vi "ScriptsCore.vi"(8 "error in (no error)":errorcluster, 10 "ScriptDatabase":refnum<class "ScriptDatabase.lvclass">, 11 "ScriptsConfiguration":refnum<class "ScriptSetting.lvclass">) -> (0 "error out":errorcluster, 3 "ScriptsConfiguration out":refnum<class "ScriptSetting.lvclass">)   [LabVIEW 2015, in "ScriptSetting.lvclass"]
uses:
  <vilib>/LazyBootMenu/ScriptsConfiguration/ScriptSetting.lvclass
  <vilib>/LazyBootMenu/_Database/Implements/ScriptDatabase.lvclass
  <vilib>/LazyBootMenu/ScriptsConfiguration/Type Definitions/Main Controls and VI Ref in ScriptsConfiguration.ctl
  <vilib>/LazyBootMenu/QDSearchList/QDDialogList.lvclass
  <vilib>/LazyBootMenu/ScriptsConfiguration/ScriptSetting.lvclass/ScriptSetting.ctl
  <vilib>/addons/database/Auxilliary.llb/DB Tools Column Info.ctl
  <vilib>/addons/database/Auxilliary.llb/DB Tools DataTypes.ctl
  <vilib>/LazyBootMenu/_Database/Implements/ScriptDatabase.lvclass/ScriptDatabase.ctl
  <vilib>/Utility/error.llb/Error Cluster From Error Code.vi
  <vilib>/ErrorRing/Error Ring.xnode
  <vilib>/LazyBootMenu/_Database/Ancestor/DatabaseAPI.lvclass
  <vilib>/addons/database/NI_Database_API.lvlib
panel:
  in  "Operation Tab":enum32{"QDFunctions", "Setting", "Options"}(tab)
  in  "Remove Select Shortcut(s)":bool
  in  "Add":bool
  in  "QD Function Full Name":string(combo)
  in  "QDAcroynm":string
  in  "QDFunction Shortcuts":i32[](listbox)
  in  "Import Shortcuts Configuration File":bool
  in  "QDFunction Library Path":path
  in  "Fresh":bool caption="Fresh QD Library"
  in  "Restore":bool
  in  "Stop":bool
  # "Add Shortcuts"
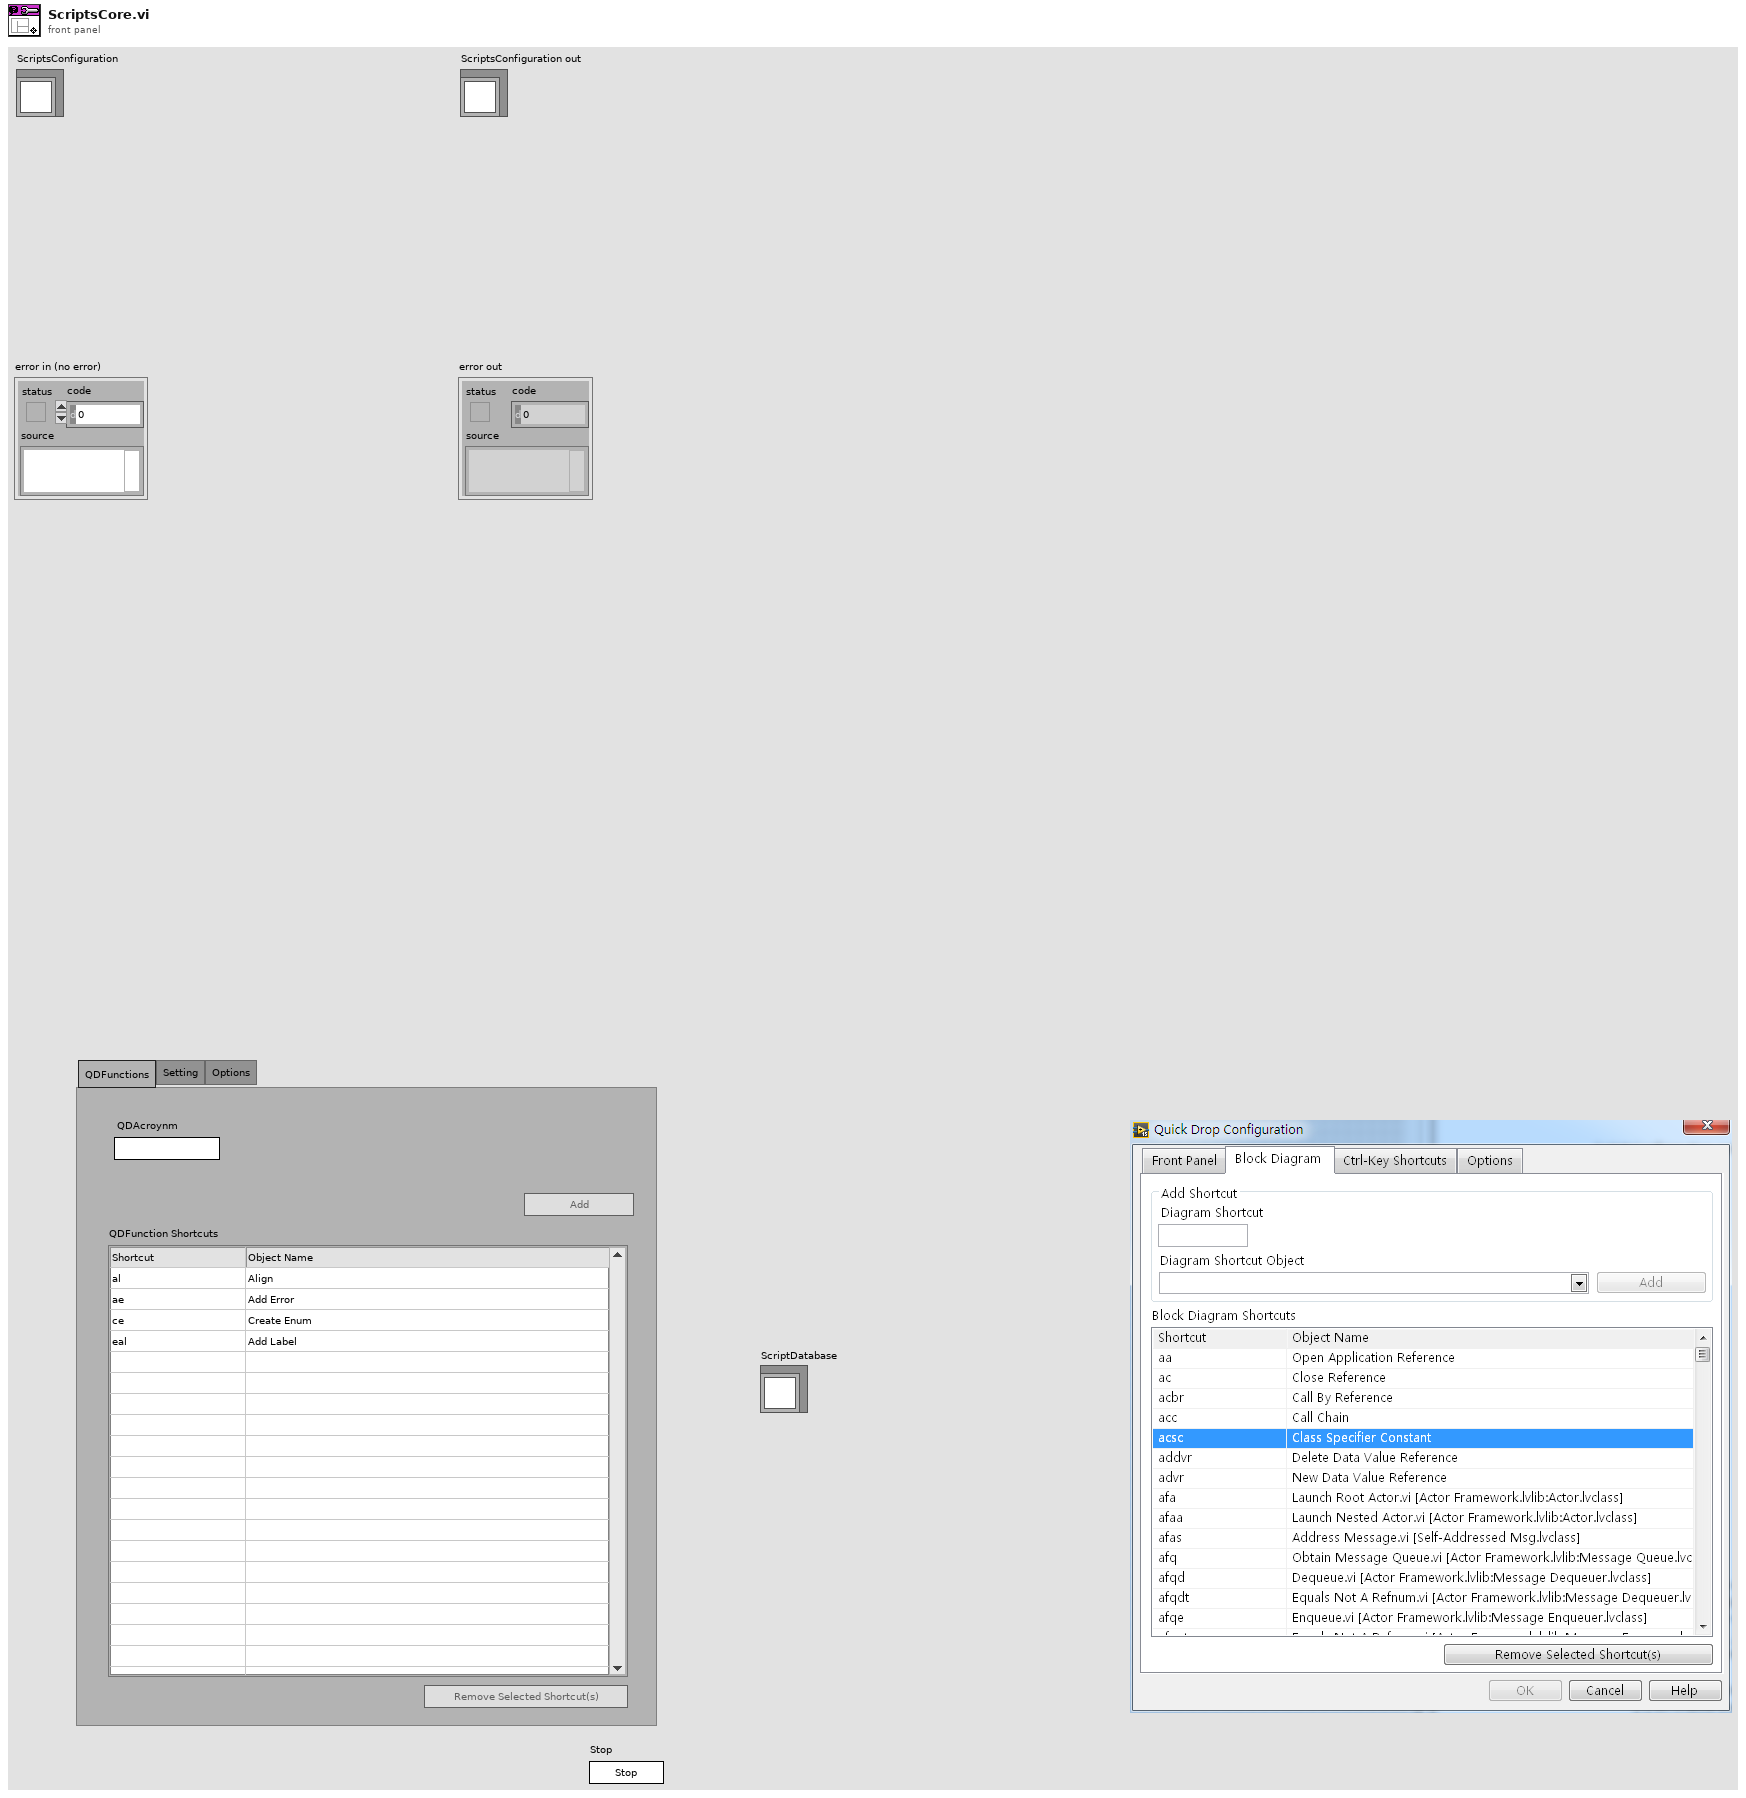
[diagram p1: front panel]
types:
  T1 = typedef "ScriptSetting.lvclass/Main Controls and VI Ref in ScriptsConfiguration.ctl" = cluster{"Fresh":refnum<vi>, "QDFunction Shortcuts":refnum<vi>, "QDAcroynm":refnum<vi>, "Import Shortcuts Configuration File":refnum<vi>, "Operation Tab":refnum<vi>, "QDFunction Library Path":refnum<vi>, "QD Function Full Name":refnum<vi>, "This VI":refnum<vi>}
  T2 = typedef "NI_Database_API.lvlib/DB Tools Column Info.ctl" = cluster{"column name":string, "data type":T3, "size":i32, "allow null?":bool}
  T3 = typedef "NI_Database_API.lvlib/DB Tools DataTypes.ctl" = enum16{"String", "Long (I32)", "Single (SGL)", "Double (DBL)", "Date/Time", "Binary"}
  T4 = enum8{"Enabled", "Disabled", "Disabled and Grayed Out"}
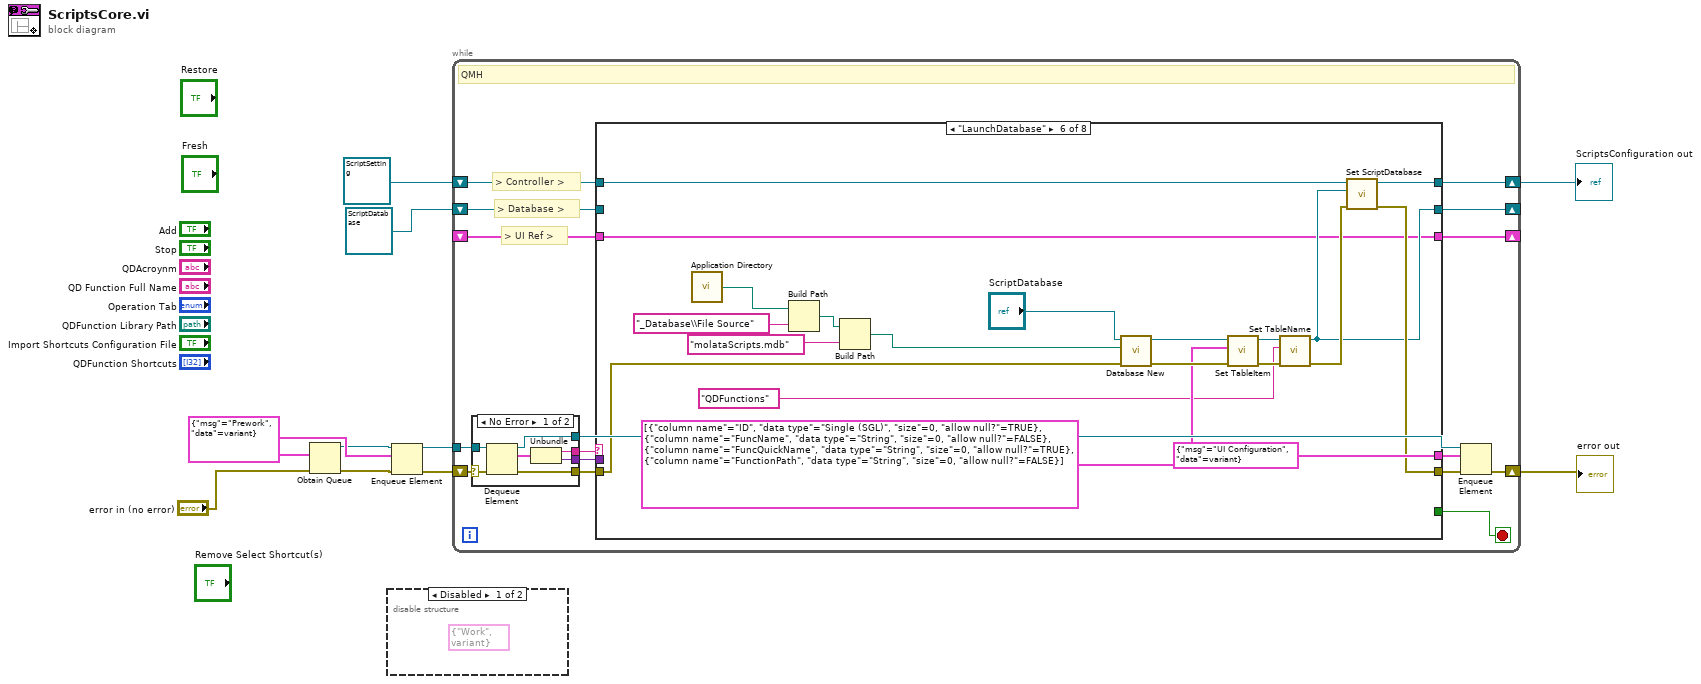
[diagram p0: block diagram]
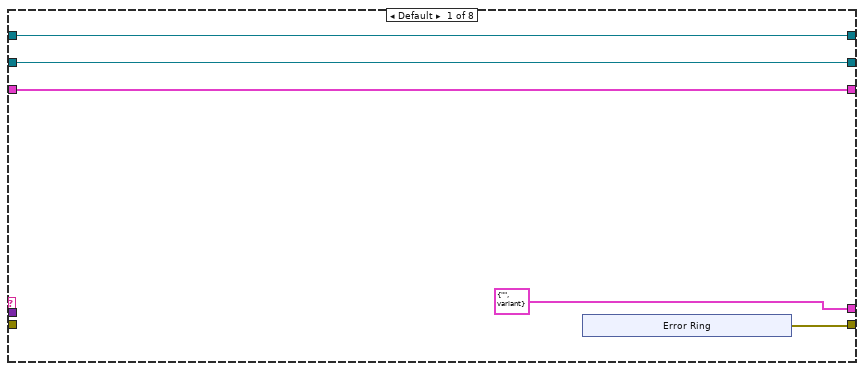
[diagram p3: hidden frame]
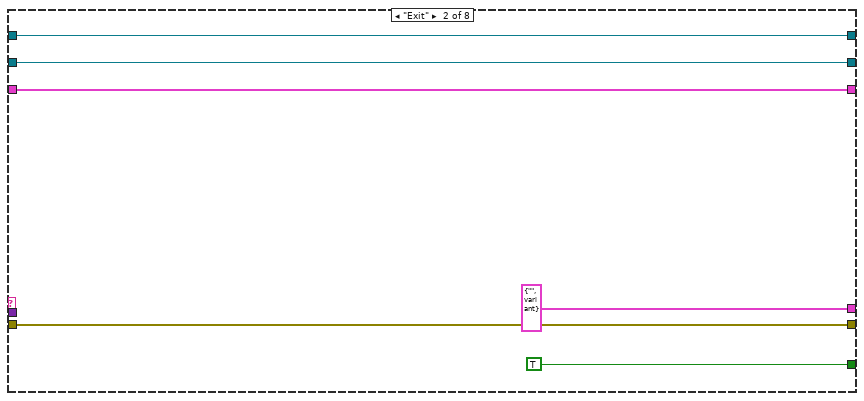
[diagram p4: hidden frame]
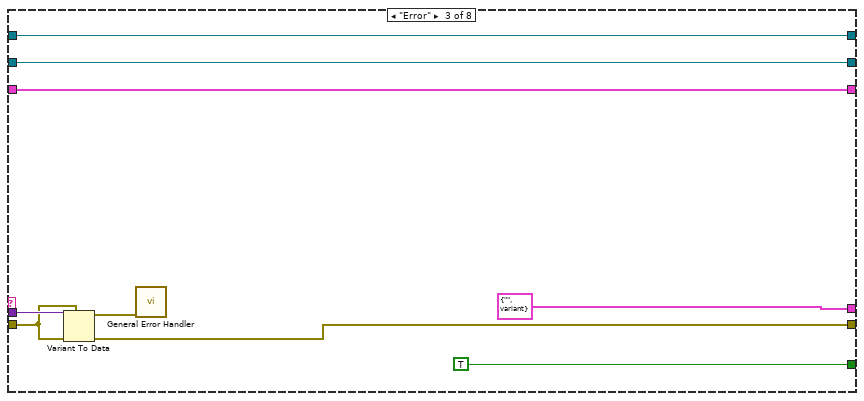
[diagram p5: hidden frame]
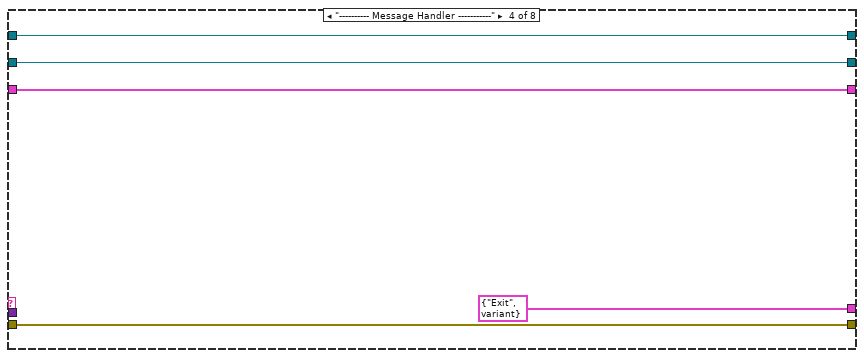
[diagram p6: hidden frame]
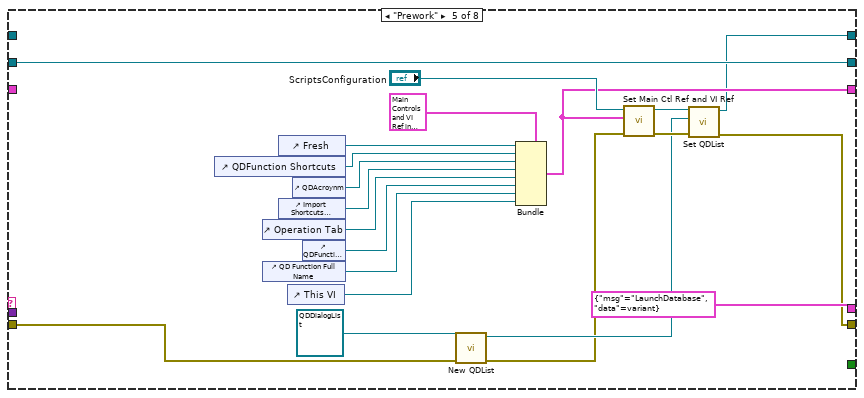
[diagram p7: hidden frame]
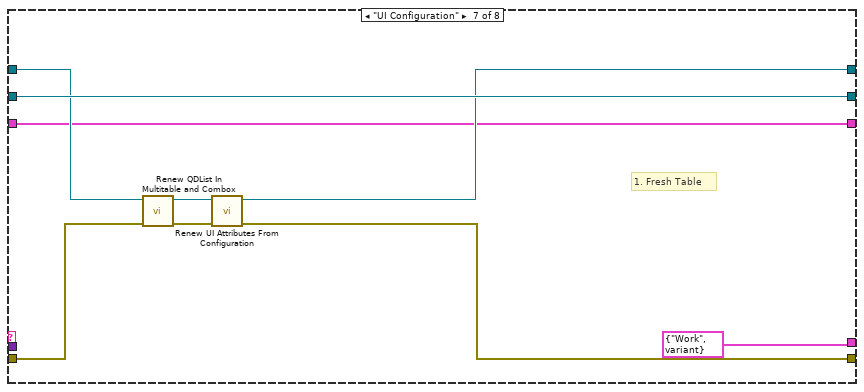
[diagram p8: hidden frame]
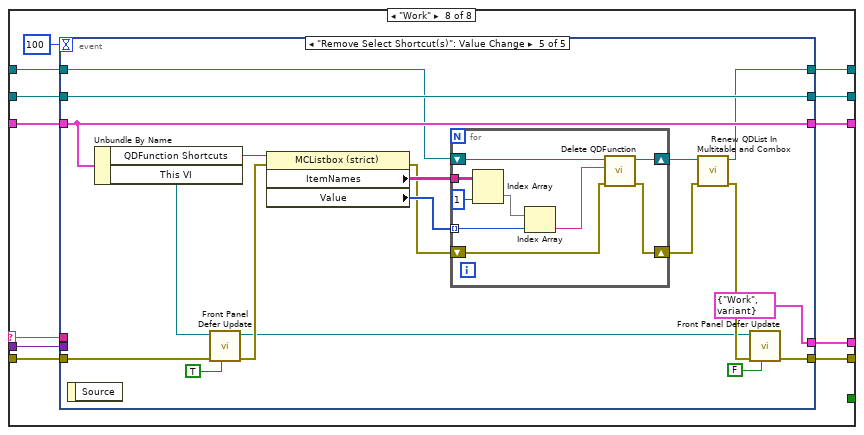
[diagram p9: hidden frame]
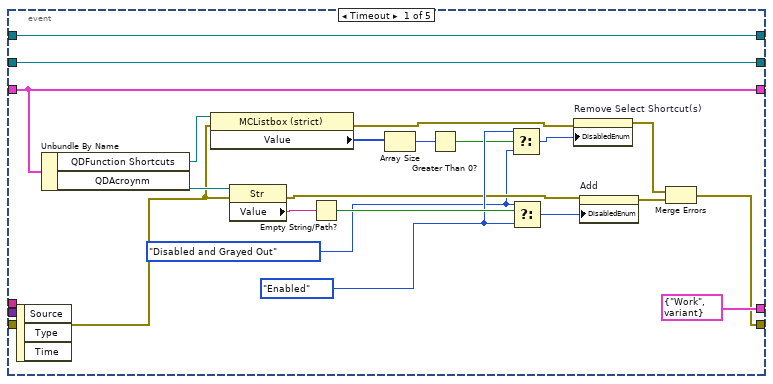
[diagram p10: hidden frame]
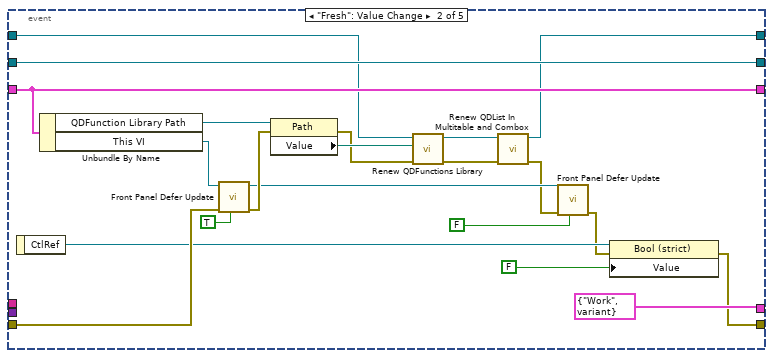
[diagram p11: hidden frame]
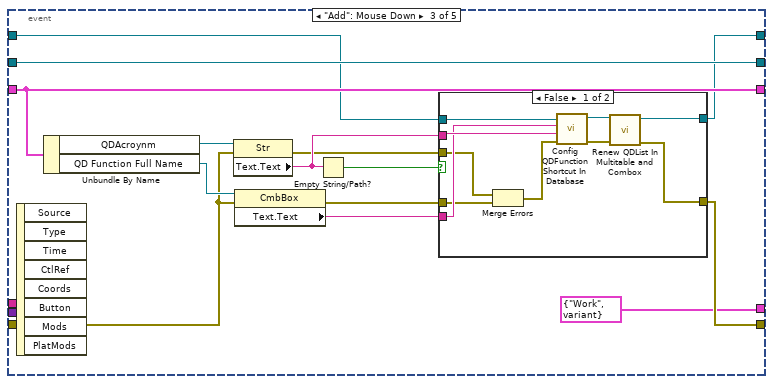
[diagram p12: hidden frame]
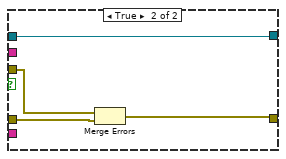
[diagram p13: hidden frame]
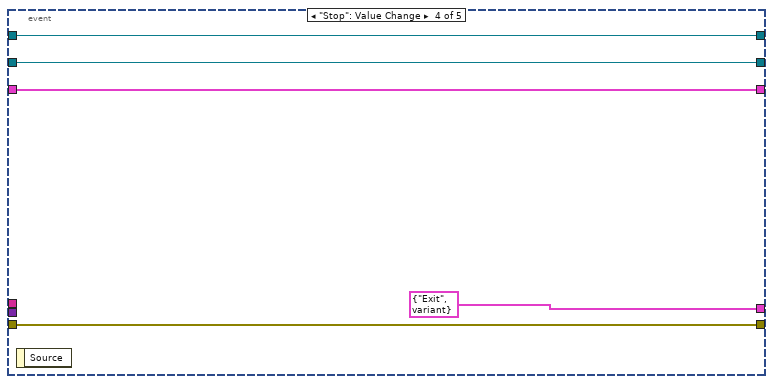
[diagram p14: hidden frame]
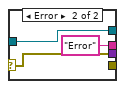
[diagram p15: hidden frame]
diagram:
  w8 = cluster{"msg":string, "data":variant} {"msg"="Prework", "data"=variant}
  n1 = Obtain Queue(element data type=w8, error in (no error)="error in (no error)") -> (queue out=w6:refnum<queue>, error out=w7:errorcluster)  [unwired: 3 in, 1 out]
  n2 = disable-structure shown="Disabled" {
    frame Disabled {
      (unwired) cluster{"msg":string, "data":variant} {"msg"="Work", "data"=variant}
    }
    frame Enabled {
    }
  }
  n3 = Enqueue Element(queue=w6, element=w8, error in (no error)=w7) -> (queue out=w9:refnum<queue>, error out=w10:errorcluster)  [unwired: 1 in, 1 out]
  n4 = while {
    tunnel: w9 -> [w25]
    shift-right: [w20] -> w1
    shift-left: w10 -> [w26]
    shift-right: [w15] -> _
    shift-left: refnum<class "ScriptDatabase.lvclass"> refnum ("ScriptDatabase out") -> [w13]
    shift-right: [w14] -> w2
    shift-left: refnum<class "ScriptSetting.lvclass"> refnum ("ScriptsConfiguration") -> [w16]
    shift-right: [w12] -> _
    shift-left: _ -> [w11]
    stop <- w17 stop-if-true
    # "> UI Ref >"
    # "> Database >"
    # "> Controller >"
    # "QMH"
    n5 = case shown="No Error" w26 {
      selector: w26 -> [w227 w231]
      tunnel: w25 -> [w228 w229]
      tunnel: [w226 _] -> w24
      tunnel: [w224 "Error" ("msg")] -> w23
      tunnel: [w223 w231] -> w22
      tunnel: [w222 w229] -> w19
      frame No Error {
        n6 = Dequeue Element(queue=w228, error in (no error)=w227) -> (queue out=w222:refnum<queue>, element=w225:cluster{"msg":string, "data":variant}, error out=w226:errorcluster)  [unwired: 1 in, 1 out]
        n7 = Unbundle(w225) -> ("msg"=w224:string, "data"=w223:variant)
      }
      frame Error {
      }
    }
    n8 = case shown="\"LaunchDatabase\"" w23 {
      selector: w23 -> [_ _ _ _ _ _ _ w116]
      tunnel: w24 -> [_ w42 w50 w56 w60 w84 w103 w118]
      tunnel: w22 -> [_ _ w51 _ _ _ _ w117]
      tunnel: [w31 w42 w48 w56 w58 w80 w100 w115] -> w21
      tunnel: [cluster{"msg":string, "data":variant} {"msg"="", "data"=variant} cluster{"msg":string, "data":variant} {"msg"="", "data"=variant} cluster{"msg":string, "data":variant} {"msg"="", "data"=variant} cluster{"msg":string, "data":variant} {"msg"="Exit", "data"=variant} cluster{"msg":string, "data":variant} {"msg"="LaunchDatabase", "data"=variant} cluster{"msg":string, "data":variant} {"msg"="UI Configuration", "data"=variant} cluster{"msg":string, "data":variant} {"msg"="Work", "data"=variant} w114] -> w18
      tunnel: [_ TRUE TRUE _ _ _ _ _] -> w17
      tunnel: w16 -> [w29 w39 w45 w54 _ w83 w104 w113]
      tunnel: [w28 w38 w44 w53 w76 w79 w106 w110] -> w15
      tunnel: [w29 w39 w45 w54 w57 w82 w99 w111] -> w14
      tunnel: w13 -> [w28 w38 w44 w53 w76 _ w106 w112]
      tunnel: [w27 w37 w43 w52 w65 w78 w98 w108] -> w12
      tunnel: w11 -> [w27 w37 w43 w52 _ w78 w98 w109]
      frame Default {
        n9 = xnode "Error Ring"() -> ("error out"=w31:errorcluster)
      }
      frame "Exit" {
      }
      frame "Error" {
        n10 = Variant To Data(error in=w50, type=w50, Variant=w51) -> (data=w49:errorcluster, error out=w48:errorcluster)
        n11 = call <vilib>:"General Error Handler.vi"("error in (no error)"=w49) -> ()  [unwired: 10 in, 5 out]
      }
      frame "---------- Message Handler -----------" {
      }
      frame "Prework" {
        n12 = control-ref of="QDFunction Shortcuts"() -> (w74:refnum<vi>)
        n13 = control-ref of="Operation Tab"() -> (w71:refnum<vi>)
        n14 = control-ref of="QD Function Full Name"() -> (w69:refnum<vi>)
        n15 = control-ref of="Fresh"() -> (w75:refnum<vi>)
        n16 = control-ref of="Import Shortcuts Configuration File"() -> (w72:refnum<vi>)
        n17 = control-ref of="This VI"() -> (w68:refnum<vi>)
        n18 = control-ref of="QDAcroynm"() -> (w73:refnum<vi>)
        n19 = control-ref of="QDFunction Library Path"() -> (w70:refnum<vi>)
        n20 = call <vilib>:"New QDList.vi"("error in (no error)"=w60, "QDDialogList in"=refnum<class "QDDialogList.lvclass"> refnum ("QDDialogList")) -> ("error out"=w59:errorcluster, "QDDialogList out"=w61:refnum<class "QDDialogList.lvclass">)  [unwired: 8 in]
        n21 = Bundle(cluster=T1 {"Fresh"=refnum, "QDFunction Shortcuts"=refnum, "QDAcroynm"=refnum, "Import Shortcuts Configuration File"=refnum, "Operation Tab"=refnum, "QDFunction Library Path"=refnum, "QD Function Full Name"=refnum, "This VI"=refnum} ("Main Ctl Ref and VI Ref"), "Fresh"=w75, "QDFunction Shortcuts"=w74, "QDAcroynm"=w73, "Import Shortcuts Configuration File"=w72, "Operation Tab"=w71, "QDFunction Library Path"=w70, "QD Function Full Name"=w69, "This VI"=w68) -> (w65:T1)
        n22 = call <vilib>:"Set Main Ctl Ref and VI Ref.vi"("error in (no error)"=w59, "Main Ctl and VI Ref"=w65, "ScriptSetting in"="ScriptsConfiguration") -> ("error out"=w63:errorcluster, "ScriptSetting out"=w64:refnum<class "ScriptSetting.lvclass">)  [unwired: 7 in]
        n23 = call <vilib>:"Set QDList.vi"("error in (no error)"=w63, "QDDialogList"=w61, "ScriptSetting in"=w64) -> ("error out"=w58:errorcluster, "ScriptSetting out"=w57:refnum<class "ScriptSetting.lvclass">)  [unwired: 7 in]
      }
      frame "LaunchDatabase" {
        n24 = call <vilib>:"Application Directory.vi"() -> ("Application Directory"=w89:path)
        n25 = Build Path(base path=w89, name or relative path="_Database\\File Source") -> (appended path=w91:path)
        n26 = Build Path(base path=w91, name or relative path="molataScripts.mdb") -> (appended path=w93:path)
        n27 = call <vilib>:"Database New.vi"("error in (no error)"=w84, "Database File Path"=w93, "object in"="ScriptDatabase") -> ("error out"=w97:errorcluster, "object out"=w96:refnum<class "ScriptDatabase.lvclass">)  [unwired: 7 in]
        n28 = call <vilib>:"Set TableItem.vi"("error in (no error)"=w97, "TableItem"=T2[] [{"column name"="ID", "data type"=enum."Single (SGL)", "size"=0, "allow null?"=TRUE}, {"column name"="FuncName", "data type"=enum."String", "size"=0, "allow null?"=FALSE}, {"column name"="FuncQuickName", "data type"=enum."String", "size"=0, "allow null?"=TRUE}, {"column name"="FunctionPath", "data type"=enum."String", "size"=0, "allow null?"=FALSE}] ("column information"), "ScriptDatabase in"=w96) -> ("error out"=w95:errorcluster, "ScriptDatabase out"=w94:refnum<class "ScriptDatabase.lvclass">)  [unwired: 7 in]
        n29 = call <vilib>:"Set TableName.vi"("error in (no error)"=w95, "TableName"="QDFunctions" ("Table"), "ScriptDatabase in"=w94) -> ("error out"=w81:errorcluster, "ScriptDatabase out"=w79:refnum<class "ScriptDatabase.lvclass">)  [unwired: 7 in]
        n30 = call <vilib>:"Set ScriptDatabase.vi"("error in (no error)"=w81, "ScriptDatabase"=w79, "ScriptsConfiguration in"=w83) -> ("error out"=w80:errorcluster, "ScriptsConfiguration out"=w82:refnum<class "ScriptSetting.lvclass">)  [unwired: 7 in]
      }
      frame "UI Configuration" {
        # "1. Fresh Table"
        n31 = call <vilib>:"Renew QDList In Multitable and Combox.vi"("error in (no error)"=w103, "ScriptsConfiguration in"=w104) -> ("error out"=w101:errorcluster, "ScriptsConfiguration out"=w102:refnum<class "ScriptSetting.lvclass">)  [unwired: 8 in]
        n32 = call <vilib>:"Renew UI Attributes From Configuration.vi"("error in (no error)"=w101, "ScriptsConfiguration in"=w102) -> ("error out"=w100:errorcluster, "ScriptsConfiguration out"=w99:refnum<class "ScriptSetting.lvclass">)  [unwired: 8 in]
      }
      frame "Work" {
        n33 = event shown="[4] \"Remove Select Shortcut(s)\": Value Change" {
          selector: _ -> [_ _ _ _ _]
          dyn-events: _ -> [_ _ _ _ _]
          timeout: 100 -> [_ _ _ _ _]
          tunnel: w118 -> [w130 w151 w167 w193 w200]
          tunnel: w117 -> [_ _ _ _ _]
          tunnel: w116 -> [_ _ _ _ _]
          tunnel: [w123 w141 w163 w193 w197] -> w115
          tunnel: [cluster{"msg":string, "data":variant} {"msg"="Work", "data"=variant} cluster{"msg":string, "data":variant} {"msg"="Work", "data"=variant} cluster{"msg":string, "data":variant} {"msg"="Work", "data"=variant} cluster{"msg":string, "data":variant} {"msg"="Exit", "data"=variant} cluster{"msg":string, "data":variant} {"msg"="Work", "data"=variant}] -> w114
          tunnel: w113 -> [w137 w157 w170 w191 w209]
          tunnel: w112 -> [w138 w160 w174 w190 w212]
          tunnel: [w137 w153 w161 w191 w203] -> w111
          tunnel: [w138 w160 w174 w190 w212] -> w110
          tunnel: w109 -> [w136 w159 w173 w189 w211]
          tunnel: [w136 w159 w173 w189 w211] -> w108
          event Timeout {
            w128 = T4."Enabled" ("Disabled")
            w122 = T4."Disabled and Grayed Out" ("Disabled")
            n34 = event-data() -> ()  [unwired: 1 in, 3 out]
            n35 = Unbundle By Name(w136) -> ("QDFunction Shortcuts"=w131:refnum<vi>, "QDAcroynm"=w135:refnum<vi>)
            n36 = property class="MCListbox (strict)"(reference=w131, error in=w130) -> (error out=w127:errorcluster, "Value"=w121:i32[])  [unwired: 1 out]
            n37 = property class="Str"(reference=w135, error in=w130) -> (error out=w126:errorcluster, "Value"=w134:string)  [unwired: 1 out]
            n38 = Empty String/Path?(string/path=w134) -> (empty?=w133:bool)
            n39 = Array Size(array=w121) -> (size(s)=w120:i32)
            n40 = Greater Than 0?(x=w120) -> (x > 0?=w119:bool)
            n41 = Select(t=w128, s=w119, f=w122) -> (s? t:f=w129:T4)
            n42 = Select(t=w122, s=w133, f=w128) -> (s? t:f=w132:T4)
            n43 = property on="Remove Select Shortcut(s)" class="Bool"(error in=w127, "DisabledEnum"=w129) -> (error out=w124:errorcluster)  [unwired: 1 in, 1 out]
            n44 = property on="Add" class="Bool (strict)"(error in=w126, "DisabledEnum"=w132) -> (error out=w125:errorcluster)  [unwired: 1 in, 1 out]
            n45 = Merge Errors(w124, w125) -> (w123:errorcluster)
          }
          event "Fresh": Value Change {
            n46 = event-data() -> ("CtlRef"=w143:refnum<vi>)  [unwired: 1 in]
            n47 = Unbundle By Name(w159) -> ("QDFunction Library Path"=w158:refnum<vi>, "This VI"=w152:refnum<vi>)
            n48 = call <userlib>:"Front Panel Defer Update.vi"("Defer Panel Updates(False)"=TRUE, "error in (no error)"=w151, "This VI"=w152) -> ("error out"=w150:errorcluster, "This VI Out"=w148:refnum<vi>)  [unwired: 7 in]
            n49 = property class="Path"(reference=w158, error in=w150) -> (error out=w155:errorcluster, "Value"=w156:path)  [unwired: 1 out]
            n50 = call <vilib>:"Renew QDFunctions Library.vi"("error in (no error)"=w155, "QDFunction Path"=w156, "ScriptSetting in"=w157) -> ("error out"=w144:errorcluster, "ScriptSetting out"=w145:refnum<class "ScriptSetting.lvclass">)  [unwired: 7 in]
            n51 = call <vilib>:"Renew QDList In Multitable and Combox.vi"("error in (no error)"=w144, "ScriptsConfiguration in"=w145) -> ("error out"=w147:errorcluster, "ScriptsConfiguration out"=w153:refnum<class "ScriptSetting.lvclass">)  [unwired: 8 in]
            n52 = call <userlib>:"Front Panel Defer Update.vi"("Defer Panel Updates(False)"=FALSE, "error in (no error)"=w147, "This VI"=w148) -> ("error out"=w142:errorcluster)  [unwired: 7 in, 1 out]
            n53 = property class="Bool (strict)"(reference=w143, error in=w142, "Value"=FALSE) -> (error out=w141:errorcluster)  [unwired: 1 out]
          }
          event "Add": Mouse Down {
            n54 = event-data() -> ()  [unwired: 1 in, 8 out]
            n55 = Unbundle By Name(w173) -> ("QDAcroynm"=w172:refnum<vi>, "QD Function Full Name"=w168:refnum<vi>)
            n56 = property class="Str"(reference=w172, error in=w167) -> (error out=w165:errorcluster, "Text.Text"=w169:string)  [unwired: 1 out]
            n57 = property class="CmbBox"(reference=w168, error in=w167) -> (error out=w164:errorcluster, "Text.Text"=w166:string)  [unwired: 1 out]
            n58 = Empty String/Path?(string/path=w169) -> (empty?=w171:bool)
            n59 = case shown="False" w171 {
              tunnel: w170 -> [w184 w188]
              tunnel: w169 -> [w183 _]
              tunnel: w166 -> [w182 _]
              tunnel: w165 -> [w180 w186]
              tunnel: w164 -> [w181 w187]
              tunnel: [w176 w185] -> w163
              tunnel: [w175 w188] -> w161
              frame False {
                n60 = Merge Errors(w180, w181) -> (w179:errorcluster)
                n61 = call <vilib>:"Config QDFunction Shortcut In Database.vi"("error in (no error)"=w179, "QDShortcut"=w183, "QDFullName"=w182, "ScriptSetting in"=w184) -> ("error out"=w177:errorcluster, "ScriptSetting out"=w178:refnum<class "ScriptSetting.lvclass">)  [unwired: 6 in]
                n62 = call <vilib>:"Renew QDList In Multitable and Combox.vi"("error in (no error)"=w177, "ScriptsConfiguration in"=w178) -> ("error out"=w176:errorcluster, "ScriptsConfiguration out"=w175:refnum<class "ScriptSetting.lvclass">)  [unwired: 8 in]
              }
              frame True {
                n63 = Merge Errors(w186, w187) -> (w185:errorcluster)
              }
            }
          }
          event "Stop": Value Change {
            n64 = event-data() -> ()  [unwired: 1 in, 1 out]
          }
          event "Remove Select Shortcut(s)": Value Change {
            n65 = event-data() -> ()  [unwired: 1 in, 1 out]
            n66 = Unbundle By Name(w211) -> ("QDFunction Shortcuts"=w210:refnum<vi>, "This VI"=w201:refnum<vi>)
            n67 = call <userlib>:"Front Panel Defer Update.vi"("Defer Panel Updates(False)"=TRUE, "error in (no error)"=w200, "This VI"=w201) -> ("error out"=w199:errorcluster, "This VI Out"=w196:refnum<vi>)  [unwired: 7 in]
            n68 = property class="MCListbox (strict)"(reference=w210, error in=w199) -> (error out=w206:errorcluster, "ItemNames"=w208:string[][], "Value"=w207:i32[])  [unwired: 1 out]
            n69 = for {
              tunnel: w208 -> [w219]
              tunnel: w207 -> [w220] mode=indexing
              shift-right: [w215] -> w204
              shift-left: w206 -> [w216]
              shift-right: [w214] -> w205
              shift-left: w209 -> [w221]
              n70 = Index Array(array=w219, index (col)=1 ("disabled index (col)")) -> (element=w218:string[])  [unwired: 1 in]
              n71 = Index Array(array=w218, index=w220) -> (element=w217:string)
              n72 = call <vilib>:"Delete QDFunction.vi"("error in (no error)"=w216, "QDFullName(\"\")"=w217, "ScriptSetting in"=w221) -> ("error out"=w215:errorcluster, "ScriptSetting out"=w214:refnum<class "ScriptSetting.lvclass">)  [unwired: 7 in]
            }
            n73 = call <vilib>:"Renew QDList In Multitable and Combox.vi"("error in (no error)"=w204, "ScriptsConfiguration in"=w205) -> ("error out"=w198:errorcluster, "ScriptsConfiguration out"=w203:refnum<class "ScriptSetting.lvclass">)  [unwired: 8 in]
            n74 = call <userlib>:"Front Panel Defer Update.vi"("Defer Panel Updates(False)"=FALSE, "error in (no error)"=w198, "This VI"=w196) -> ("error out"=w197:errorcluster)  [unwired: 7 in, 1 out]
          }
        }
      }
    }
    n75 = Enqueue Element(queue=w19, element=w18, error in (no error)=w21) -> (error out=w20:errorcluster)  [unwired: 1 in, 2 out]
  }
  "error out" <- w1
  "ScriptsConfiguration out" <- w2
